vi "S4GUI_001.vi"() -> ()   [LabVIEW 2018] (continued)
            n3129 = call-dynamic "Read State Machine.vi"("error in (no error)"=w7702, "Device in"=w7704) -> ("error out"=w7725:errorcluster, "State Machine.lvclass"=w7726:refnum<class "State Machine.lvclass">, "Device out"=w7722:refnum<class "Channel.lvclass">)  [unwired: 7 in]
            n3130 = call "Next State.vi"("error in (no error)"=w7725, "New_State"=u32 35, "State Machine in"=w7726) -> ("error out"=w7720:errorcluster, "State Machine out"=w7723:refnum<class "State Machine.lvclass">)  [unwired: 7 in]
            n3131 = call-dynamic "Write State Machine.vi"("error in (no error)"=w7720, "State Machine.lvclass"=w7723, "Device in"=w7722) -> ("error out"=w7716:errorcluster, "Device out"=w7715:refnum<class "Channel.lvclass">)  [unwired: 7 in]
            n3132 = call-dynamic "Write Channel.vi"("error in (no error)"=w7716, "Channel.lvclass"=w7715, "Acquisition in"=w7721) -> ("error out"=w7717:errorcluster, "Acquisition out"=w7719:refnum<class "Acquisition.lvclass">)  [unwired: 7 in]
            n3133 = call-dynamic "Write AcquisitionC.vi"("error in (no error)"=w7717, "Acquisition.lvclass"=w7719, "S4ACS_GUI in"=w7718) -> ("error out"=w7712:errorcluster, "S4ACS_GUI out"=w7711:refnum<class "S4GUI.lvclass">)  [unwired: 7 in]
          }
        }
      }
      event "Set Temp 4": Value Change {
        n3134 = event-data() -> ("NewVal"=w7729:bool)  [unwired: 1 in]
        n3135 = case shown="True" w7729 {
          tunnel: w7733 -> [w7735 w7749]
          tunnel: w7732 -> [w7734 w7748]
          tunnel: [w7734 w7747] -> w7731
          tunnel: [w7735 w7746] -> w7730
          frame False {
          }
          frame True {
            n3136 = call-dynamic "Read AcquisitionD.vi"("error in (no error)"=w7748, "S4ACS_GUI in"=w7749) -> ("error out"=w7762:errorcluster, "Acquisition.lvclass"=w7763:refnum<class "Acquisition.lvclass">, "S4ACS_GUI out"=w7753:refnum<class "S4GUI.lvclass">)  [unwired: 7 in]
            n3137 = call-dynamic "Read Channel.vi"("error in (no error)"=w7762, "Acquisition in"=w7763) -> ("error out"=w7744:errorcluster, "Channel.lvclass"=w7745:refnum<class "Channel.lvclass">, "Acquisition out"=w7756:refnum<class "Acquisition.lvclass">)  [unwired: 7 in]
            n3138 = call-dynamic "Read Interface.vi"("error in (no error)"=w7744, "Channel in"=w7745) -> ("error out"=w7742:errorcluster, "Interface.lvclass"=w7743:refnum<class "Interface.lvclass">, "Channel out"=w7740:refnum<class "Channel.lvclass">)  [unwired: 7 in]
            n3139 = call-dynamic "Write Temperature.vi"("error in (no error)"=w7742, "Temperature"="Target Temp 4", "Interface in"=w7743) -> ("error out"=w7738:errorcluster, "Interface out"=w7741:refnum<class "Interface.lvclass">)  [unwired: 7 in]
            n3140 = call-dynamic "Write Interface.vi"("error in (no error)"=w7738, "Interface.lvclass"=w7741, "Channel in"=w7740) -> ("error out"=w7737:errorcluster, "Channel out"=w7739:refnum<class "Channel.lvclass">)  [unwired: 7 in]
            n3141 = call-dynamic "Read State Machine.vi"("error in (no error)"=w7737, "Device in"=w7739) -> ("error out"=w7760:errorcluster, "State Machine.lvclass"=w7761:refnum<class "State Machine.lvclass">, "Device out"=w7757:refnum<class "Channel.lvclass">)  [unwired: 7 in]
            n3142 = call "Next State.vi"("error in (no error)"=w7760, "New_State"=u32 35, "State Machine in"=w7761) -> ("error out"=w7755:errorcluster, "State Machine out"=w7758:refnum<class "State Machine.lvclass">)  [unwired: 7 in]
            n3143 = call-dynamic "Write State Machine.vi"("error in (no error)"=w7755, "State Machine.lvclass"=w7758, "Device in"=w7757) -> ("error out"=w7751:errorcluster, "Device out"=w7750:refnum<class "Channel.lvclass">)  [unwired: 7 in]
            n3144 = call-dynamic "Write Channel.vi"("error in (no error)"=w7751, "Channel.lvclass"=w7750, "Acquisition in"=w7756) -> ("error out"=w7752:errorcluster, "Acquisition out"=w7754:refnum<class "Acquisition.lvclass">)  [unwired: 7 in]
            n3145 = call-dynamic "Write AcquisitionD.vi"("error in (no error)"=w7752, "Acquisition.lvclass"=w7754, "S4ACS_GUI in"=w7753) -> ("error out"=w7747:errorcluster, "S4ACS_GUI out"=w7746:refnum<class "S4GUI.lvclass">)  [unwired: 7 in]
          }
        }
      }
      event "Avança Estado": Value Change {
        n3146 = event-data() -> ()  [unwired: 1 in, 4 out]
        n3147 = call-dynamic "Read Sync Box.lvclass.vi"("error in (no error)"=w7772, "SPARC4_AC in"=w7773) -> ("error out"=w7785:errorcluster, "Sync Box.lvclass"=w7786:refnum<class "Sync Box.lvclass">, "SPARC4_AC out"=w7777:refnum<class "S4GUI.lvclass">)  [unwired: 7 in]
        n3148 = call-dynamic "Read Trigger.lvclass.vi"("error in (no error)"=w7785, "Sync Box in"=w7786) -> ("error out"=w7783:errorcluster, "Trigger.lvclass"=w7784:refnum<class "Trigger.lvclass">, "Sync Box out"=w7780:refnum<class "Sync Box.lvclass">)  [unwired: 7 in]
        n3149 = call-dynamic "Read State Machine.vi"("error in (no error)"=w7783, "Device in"=w7784) -> ("error out"=w7769:errorcluster, "State Machine.lvclass"=w7770:refnum<class "State Machine.lvclass">, "Device out"=w7781:refnum<class "Trigger.lvclass">)  [unwired: 7 in]
        n3150 = call-dynamic "Read State.vi"("error in (no error)"=w7769, "State Machine in"=w7770) -> ("error out"=w7765:errorcluster, "State"=w7768:i32, "State Machine out"=w7766:refnum<class "State Machine.lvclass">)  [unwired: 7 in]
        n3151 = Increment(x=w7768) -> (x+1=w7767:i32)
        n3152 = call "Next State.vi"("error in (no error)"=w7765, "New_State"=w7767, "State Machine in"=w7766) -> ("error out"=w7779:errorcluster, "State Machine out"=w7782:refnum<class "State Machine.lvclass">)  [unwired: 7 in]
        n3153 = call-dynamic "Write State Machine.vi"("error in (no error)"=w7779, "State Machine.lvclass"=w7782, "Device in"=w7781) -> ("error out"=w7775:errorcluster, "Device out"=w7774:refnum<class "Trigger.lvclass">)  [unwired: 7 in]
        n3154 = call-dynamic "Write Trigger.lvclass.vi"("error in (no error)"=w7775, "Trigger.lvclass"=w7774, "Sync Box in"=w7780) -> ("error out"=w7776:errorcluster, "Sync Box out"=w7778:refnum<class "Sync Box.lvclass">)  [unwired: 7 in]
        n3155 = call-dynamic "Write Sync Box.lvclass.vi"("error in (no error)"=w7776, "Sync Box.lvclass"=w7778, "SPARC4_AC in"=w7777) -> ("error out"=w7771:errorcluster, "SPARC4_AC out"=w7764:refnum<class "S4GUI.lvclass">)  [unwired: 7 in]
      }
      event "DelayA": Value Change {
        n3156 = event-data() -> ("NewVal"=w7788:string)  [unwired: 1 in, 3 out]
        n3157 = call-dynamic "Read Sync Box.lvclass.vi"("error in (no error)"=w7792, "SPARC4_AC in"=w7793) -> ("error out"=w7800:errorcluster, "Sync Box.lvclass"=w7801:refnum<class "Sync Box.lvclass">, "SPARC4_AC out"=w7797:refnum<class "S4GUI.lvclass">)  [unwired: 7 in]
        n3158 = call-dynamic "Read Trigger.lvclass.vi"("error in (no error)"=w7800, "Sync Box in"=w7801) -> ("error out"=w7789:errorcluster, "Trigger.lvclass"=w7790:refnum<class "Trigger.lvclass">, "Sync Box out"=w7799:refnum<class "Sync Box.lvclass">)  [unwired: 7 in]
        n3159 = call-dynamic "Write DelayA.vi"("error in (no error)"=w7789, "DelayA"=w7788, "Trigger in"=w7790) -> ("error out"=w7795:errorcluster, "Trigger out"=w7794:refnum<class "Trigger.lvclass">)  [unwired: 7 in]
        n3160 = call-dynamic "Write Trigger.lvclass.vi"("error in (no error)"=w7795, "Trigger.lvclass"=w7794, "Sync Box in"=w7799) -> ("error out"=w7796:errorcluster, "Sync Box out"=w7798:refnum<class "Sync Box.lvclass">)  [unwired: 7 in]
        n3161 = call-dynamic "Write Sync Box.lvclass.vi"("error in (no error)"=w7796, "Sync Box.lvclass"=w7798, "SPARC4_AC in"=w7797) -> ("error out"=w7791:errorcluster, "SPARC4_AC out"=w7787:refnum<class "S4GUI.lvclass">)  [unwired: 7 in]
      }
      event "DelayB": Value Change {
        n3162 = event-data() -> ("NewVal"=w7803:string)  [unwired: 1 in, 3 out]
        n3163 = call-dynamic "Read Sync Box.lvclass.vi"("error in (no error)"=w7807, "SPARC4_AC in"=w7808) -> ("error out"=w7815:errorcluster, "Sync Box.lvclass"=w7816:refnum<class "Sync Box.lvclass">, "SPARC4_AC out"=w7812:refnum<class "S4GUI.lvclass">)  [unwired: 7 in]
        n3164 = call-dynamic "Read Trigger.lvclass.vi"("error in (no error)"=w7815, "Sync Box in"=w7816) -> ("error out"=w7804:errorcluster, "Trigger.lvclass"=w7805:refnum<class "Trigger.lvclass">, "Sync Box out"=w7814:refnum<class "Sync Box.lvclass">)  [unwired: 7 in]
        n3165 = call-dynamic "Write DelayB.vi"("error in (no error)"=w7804, "DelayB"=w7803, "Trigger in"=w7805) -> ("error out"=w7810:errorcluster, "Trigger out"=w7809:refnum<class "Trigger.lvclass">)  [unwired: 7 in]
        n3166 = call-dynamic "Write Trigger.lvclass.vi"("error in (no error)"=w7810, "Trigger.lvclass"=w7809, "Sync Box in"=w7814) -> ("error out"=w7811:errorcluster, "Sync Box out"=w7813:refnum<class "Sync Box.lvclass">)  [unwired: 7 in]
        n3167 = call-dynamic "Write Sync Box.lvclass.vi"("error in (no error)"=w7811, "Sync Box.lvclass"=w7813, "SPARC4_AC in"=w7812) -> ("error out"=w7806:errorcluster, "SPARC4_AC out"=w7802:refnum<class "S4GUI.lvclass">)  [unwired: 7 in]
      }
      event "DelayC": Value Change {
        n3168 = event-data() -> ("NewVal"=w7818:string)  [unwired: 1 in, 3 out]
        n3169 = call-dynamic "Read Sync Box.lvclass.vi"("error in (no error)"=w7822, "SPARC4_AC in"=w7823) -> ("error out"=w7830:errorcluster, "Sync Box.lvclass"=w7831:refnum<class "Sync Box.lvclass">, "SPARC4_AC out"=w7827:refnum<class "S4GUI.lvclass">)  [unwired: 7 in]
        n3170 = call-dynamic "Read Trigger.lvclass.vi"("error in (no error)"=w7830, "Sync Box in"=w7831) -> ("error out"=w7819:errorcluster, "Trigger.lvclass"=w7820:refnum<class "Trigger.lvclass">, "Sync Box out"=w7829:refnum<class "Sync Box.lvclass">)  [unwired: 7 in]
        n3171 = call-dynamic "Write DelayC.vi"("error in (no error)"=w7819, "DelayC"=w7818, "Trigger in"=w7820) -> ("error out"=w7825:errorcluster, "Trigger out"=w7824:refnum<class "Trigger.lvclass">)  [unwired: 7 in]
        n3172 = call-dynamic "Write Trigger.lvclass.vi"("error in (no error)"=w7825, "Trigger.lvclass"=w7824, "Sync Box in"=w7829) -> ("error out"=w7826:errorcluster, "Sync Box out"=w7828:refnum<class "Sync Box.lvclass">)  [unwired: 7 in]
        n3173 = call-dynamic "Write Sync Box.lvclass.vi"("error in (no error)"=w7826, "Sync Box.lvclass"=w7828, "SPARC4_AC in"=w7827) -> ("error out"=w7821:errorcluster, "SPARC4_AC out"=w7817:refnum<class "S4GUI.lvclass">)  [unwired: 7 in]
      }
      event "DelayD": Value Change {
        n3174 = event-data() -> ("NewVal"=w7833:string)  [unwired: 1 in, 3 out]
        n3175 = call-dynamic "Read Sync Box.lvclass.vi"("error in (no error)"=w7837, "SPARC4_AC in"=w7838) -> ("error out"=w7845:errorcluster, "Sync Box.lvclass"=w7846:refnum<class "Sync Box.lvclass">, "SPARC4_AC out"=w7842:refnum<class "S4GUI.lvclass">)  [unwired: 7 in]
        n3176 = call-dynamic "Read Trigger.lvclass.vi"("error in (no error)"=w7845, "Sync Box in"=w7846) -> ("error out"=w7834:errorcluster, "Trigger.lvclass"=w7835:refnum<class "Trigger.lvclass">, "Sync Box out"=w7844:refnum<class "Sync Box.lvclass">)  [unwired: 7 in]
        n3177 = call-dynamic "Write DelayD.vi"("error in (no error)"=w7834, "DelayD"=w7833, "Trigger in"=w7835) -> ("error out"=w7840:errorcluster, "Trigger out"=w7839:refnum<class "Trigger.lvclass">)  [unwired: 7 in]
        n3178 = call-dynamic "Write Trigger.lvclass.vi"("error in (no error)"=w7840, "Trigger.lvclass"=w7839, "Sync Box in"=w7844) -> ("error out"=w7841:errorcluster, "Sync Box out"=w7843:refnum<class "Sync Box.lvclass">)  [unwired: 7 in]
        n3179 = call-dynamic "Write Sync Box.lvclass.vi"("error in (no error)"=w7841, "Sync Box.lvclass"=w7843, "SPARC4_AC in"=w7842) -> ("error out"=w7836:errorcluster, "SPARC4_AC out"=w7832:refnum<class "S4GUI.lvclass">)  [unwired: 7 in]
      }
      event "WidthA": Value Change {
        n3180 = event-data() -> ("NewVal"=w7848:string)  [unwired: 1 in, 3 out]
        n3181 = call-dynamic "Read Sync Box.lvclass.vi"("error in (no error)"=w7852, "SPARC4_AC in"=w7853) -> ("error out"=w7860:errorcluster, "Sync Box.lvclass"=w7861:refnum<class "Sync Box.lvclass">, "SPARC4_AC out"=w7857:refnum<class "S4GUI.lvclass">)  [unwired: 7 in]
        n3182 = call-dynamic "Read Trigger.lvclass.vi"("error in (no error)"=w7860, "Sync Box in"=w7861) -> ("error out"=w7849:errorcluster, "Trigger.lvclass"=w7850:refnum<class "Trigger.lvclass">, "Sync Box out"=w7859:refnum<class "Sync Box.lvclass">)  [unwired: 7 in]
        n3183 = call-dynamic "Write WidthA.vi"("error in (no error)"=w7849, "WidthA"=w7848, "Trigger in"=w7850) -> ("error out"=w7855:errorcluster, "Trigger out"=w7854:refnum<class "Trigger.lvclass">)  [unwired: 7 in]
        n3184 = call-dynamic "Write Trigger.lvclass.vi"("error in (no error)"=w7855, "Trigger.lvclass"=w7854, "Sync Box in"=w7859) -> ("error out"=w7856:errorcluster, "Sync Box out"=w7858:refnum<class "Sync Box.lvclass">)  [unwired: 7 in]
        n3185 = call-dynamic "Write Sync Box.lvclass.vi"("error in (no error)"=w7856, "Sync Box.lvclass"=w7858, "SPARC4_AC in"=w7857) -> ("error out"=w7851:errorcluster, "SPARC4_AC out"=w7847:refnum<class "S4GUI.lvclass">)  [unwired: 7 in]
      }
      event "WidthB": Value Change {
        n3186 = event-data() -> ("NewVal"=w7863:string)  [unwired: 1 in, 3 out]
        n3187 = call-dynamic "Read Sync Box.lvclass.vi"("error in (no error)"=w7867, "SPARC4_AC in"=w7868) -> ("error out"=w7875:errorcluster, "Sync Box.lvclass"=w7876:refnum<class "Sync Box.lvclass">, "SPARC4_AC out"=w7872:refnum<class "S4GUI.lvclass">)  [unwired: 7 in]
        n3188 = call-dynamic "Read Trigger.lvclass.vi"("error in (no error)"=w7875, "Sync Box in"=w7876) -> ("error out"=w7864:errorcluster, "Trigger.lvclass"=w7865:refnum<class "Trigger.lvclass">, "Sync Box out"=w7874:refnum<class "Sync Box.lvclass">)  [unwired: 7 in]
        n3189 = call-dynamic "Write WidthB.vi"("error in (no error)"=w7864, "WidthB"=w7863, "Trigger in"=w7865) -> ("error out"=w7870:errorcluster, "Trigger out"=w7869:refnum<class "Trigger.lvclass">)  [unwired: 7 in]
        n3190 = call-dynamic "Write Trigger.lvclass.vi"("error in (no error)"=w7870, "Trigger.lvclass"=w7869, "Sync Box in"=w7874) -> ("error out"=w7871:errorcluster, "Sync Box out"=w7873:refnum<class "Sync Box.lvclass">)  [unwired: 7 in]
        n3191 = call-dynamic "Write Sync Box.lvclass.vi"("error in (no error)"=w7871, "Sync Box.lvclass"=w7873, "SPARC4_AC in"=w7872) -> ("error out"=w7866:errorcluster, "SPARC4_AC out"=w7862:refnum<class "S4GUI.lvclass">)  [unwired: 7 in]
      }
      event "WidthC": Value Change {
        n3192 = event-data() -> ("NewVal"=w7878:string)  [unwired: 1 in, 3 out]
        n3193 = call-dynamic "Read Sync Box.lvclass.vi"("error in (no error)"=w7882, "SPARC4_AC in"=w7883) -> ("error out"=w7890:errorcluster, "Sync Box.lvclass"=w7891:refnum<class "Sync Box.lvclass">, "SPARC4_AC out"=w7887:refnum<class "S4GUI.lvclass">)  [unwired: 7 in]
        n3194 = call-dynamic "Read Trigger.lvclass.vi"("error in (no error)"=w7890, "Sync Box in"=w7891) -> ("error out"=w7879:errorcluster, "Trigger.lvclass"=w7880:refnum<class "Trigger.lvclass">, "Sync Box out"=w7889:refnum<class "Sync Box.lvclass">)  [unwired: 7 in]
        n3195 = call-dynamic "Write WidthC.vi"("error in (no error)"=w7879, "WidthC"=w7878, "Trigger in"=w7880) -> ("error out"=w7885:errorcluster, "Trigger out"=w7884:refnum<class "Trigger.lvclass">)  [unwired: 7 in]
        n3196 = call-dynamic "Write Trigger.lvclass.vi"("error in (no error)"=w7885, "Trigger.lvclass"=w7884, "Sync Box in"=w7889) -> ("error out"=w7886:errorcluster, "Sync Box out"=w7888:refnum<class "Sync Box.lvclass">)  [unwired: 7 in]
        n3197 = call-dynamic "Write Sync Box.lvclass.vi"("error in (no error)"=w7886, "Sync Box.lvclass"=w7888, "SPARC4_AC in"=w7887) -> ("error out"=w7881:errorcluster, "SPARC4_AC out"=w7877:refnum<class "S4GUI.lvclass">)  [unwired: 7 in]
      }
      event "WidthD": Value Change {
        n3198 = event-data() -> ("NewVal"=w7893:string)  [unwired: 1 in, 3 out]
        n3199 = call-dynamic "Read Sync Box.lvclass.vi"("error in (no error)"=w7897, "SPARC4_AC in"=w7898) -> ("error out"=w7905:errorcluster, "Sync Box.lvclass"=w7906:refnum<class "Sync Box.lvclass">, "SPARC4_AC out"=w7902:refnum<class "S4GUI.lvclass">)  [unwired: 7 in]
        n3200 = call-dynamic "Read Trigger.lvclass.vi"("error in (no error)"=w7905, "Sync Box in"=w7906) -> ("error out"=w7894:errorcluster, "Trigger.lvclass"=w7895:refnum<class "Trigger.lvclass">, "Sync Box out"=w7904:refnum<class "Sync Box.lvclass">)  [unwired: 7 in]
        n3201 = call-dynamic "Write WidthD.vi"("error in (no error)"=w7894, "WidthD"=w7893, "Trigger in"=w7895) -> ("error out"=w7900:errorcluster, "Trigger out"=w7899:refnum<class "Trigger.lvclass">)  [unwired: 7 in]
        n3202 = call-dynamic "Write Trigger.lvclass.vi"("error in (no error)"=w7900, "Trigger.lvclass"=w7899, "Sync Box in"=w7904) -> ("error out"=w7901:errorcluster, "Sync Box out"=w7903:refnum<class "Sync Box.lvclass">)  [unwired: 7 in]
        n3203 = call-dynamic "Write Sync Box.lvclass.vi"("error in (no error)"=w7901, "Sync Box.lvclass"=w7903, "SPARC4_AC in"=w7902) -> ("error out"=w7896:errorcluster, "SPARC4_AC out"=w7892:refnum<class "S4GUI.lvclass">)  [unwired: 7 in]
      }
      event "WPROT_set": Value Change {
        # "Espera até 10 x 1s = 10s\npara condition de WPROT\n ir para READY"
        n3204 = event-data() -> ()  [unwired: 1 in, 4 out]
        n3205 = call "Read Instrument.lvclass.vi"("error in (no error)"=w7928, "S4ACS_GUI in"=w7929) -> ("error out"=w7926:errorcluster, "Instrument.lvclass"=w7927:refnum<class "Instrument.lvclass">, "S4ACS_GUI out"=w7915:refnum<class "S4GUI.lvclass">)  [unwired: 7 in]
        n3206 = call "Read WPROT.vi"("error in (no error)"=w7926, "Instrument in"=w7927) -> ("error out"=w7922:errorcluster, "Opt_Selector.lvclass"=w7925:refnum<class "Opt_Selector.lvclass">, "Instrument out"=w7918:refnum<class "Instrument.lvclass">)  [unwired: 7 in]
        n3207 = call-dynamic "Read State Machine.vi"("error in (no error)"=w7922, "Device in"=w7925) -> ("error out"=w7921:errorcluster, "State Machine.lvclass"=w7924:refnum<class "State Machine.lvclass">, "Device out"=w7920:refnum<class "Opt_Selector.lvclass">)  [unwired: 7 in]
        n3208 = call "Next State.vi"("error in (no error)"=w7921, "New_State"=1, "State Machine in"=w7924) -> ("error out"=w7909:errorcluster, "State Machine out"=w7911:refnum<class "State Machine.lvclass">)  [unwired: 7 in]
        n3209 = call-dynamic "Write Timer.vi"("error in (no error)"=w7909, "Timer"=u32 10, "State Machine in"=w7911) -> ("error out"=w7908:errorcluster, "State Machine out"=w7910:refnum<class "State Machine.lvclass">)  [unwired: 7 in]
        n3210 = call-dynamic "Write State Machine.vi"("error in (no error)"=w7908, "State Machine.lvclass"=w7910, "Device in"=w7920) -> ("error out"=w7917:errorcluster, "Device out"=w7919:refnum<class "Opt_Selector.lvclass">)  [unwired: 7 in]
        n3211 = call "Write WPROT.vi"("error in (no error)"=w7917, "Opt_Selector.lvclass"=w7919, "Instrument in"=w7918) -> ("error out"=w7914:errorcluster, "Instrument out"=w7916:refnum<class "Instrument.lvclass">)  [unwired: 7 in]
        n3212 = call "Write Instrument.lvclass.vi"("error in (no error)"=w7914, "Instrument.lvclass"=w7916, "S4ACS_GUI in"=w7915) -> ("error out"=w7913:errorcluster, "S4ACS_GUI out"=w7912:refnum<class "S4GUI.lvclass">)  [unwired: 7 in]
      }
      event "TARGET NAME WPROT": Value Change {
        n3213 = event-data() -> ()  [unwired: 1 in, 1 out]
        n3214 = property on="TARGET NAME WPROT" class="Enum (strict)"() -> ("RingText.Text"=w7956:string)  [unwired: 2 in, 2 out]
        n3215 = call "Read Instrument.lvclass.vi"("error in (no error)"=w7957, "S4ACS_GUI in"=w7958) -> ("error out"=w7965:errorcluster, "Instrument.lvclass"=w7966:refnum<class "Instrument.lvclass">, "S4ACS_GUI out"=w7960:refnum<class "S4GUI.lvclass">)  [unwired: 7 in]
        n3216 = Build Array(-1.0 ("element"), 0.0 ("element"), 22.5 ("element"), 45.0 ("element"), 67.5 ("element"), 90.0 ("element"), 112.5 ("element"), 135.0 ("element"), 157.5 ("element"), 180.0 ("element"), 202.5 ("element"), 225.0 ("element"), 247.5 ("element"), 270.0 ("element"), 292.5 ("element"), 315.0 ("element"), 337.5 ("element")) -> (w7948:dbl[])
        n3217 = call "Read WPROT.vi"("error in (no error)"=w7965, "Instrument in"=w7966) -> ("error out"=w7963:errorcluster, "Opt_Selector.lvclass"=w7964:refnum<class "Opt_Selector.lvclass">, "Instrument out"=w7962:refnum<class "Instrument.lvclass">)  [unwired: 7 in]
        n3218 = call "Write target name.vi"("error in (no error)"=w7963, "target name"=w7956, "Optics in"=w7964) -> ("error out"=w7944:errorcluster, "Optics out"=w7945:refnum<class "Opt_Selector.lvclass">)  [unwired: 7 in]
        n3219 = Index Array(array=w7948, index="TARGET NAME WPROT") -> (element=w7946:dbl)
        n3220 = call "Write target.vi"("error in (no error)"=w7944, "target"=w7946, "Optics in"=w7945) -> ("error out"=w7943:errorcluster, "Optics out"=w7942:refnum<class "Opt_Selector.lvclass">)  [unwired: 7 in]
        n3221 = call "Write WPROT.vi"("error in (no error)"=w7943, "Opt_Selector.lvclass"=w7942, "Instrument in"=w7962) -> ("error out"=w7959:errorcluster, "Instrument out"=w7961:refnum<class "Instrument.lvclass">)  [unwired: 7 in]
        n3222 = call "Write Instrument.lvclass.vi"("error in (no error)"=w7959, "Instrument.lvclass"=w7961, "S4ACS_GUI in"=w7960) -> ("error out"=w7955:errorcluster, "S4ACS_GUI out"=w7930:refnum<class "S4GUI.lvclass">)  [unwired: 7 in]
      }
      event "TARGET NAME WPSEL": Value Change {
        n3223 = event-data() -> ()  [unwired: 1 in, 1 out]
        n3224 = property on="TARGET NAME WPSEL" class="Enum (strict)"() -> ("RingText.Text"=w7968:string)  [unwired: 2 in, 2 out]
        n3225 = call "Read Instrument.lvclass.vi"("error in (no error)"=w7981, "S4ACS_GUI in"=w7982) -> ("error out"=w7989:errorcluster, "Instrument.lvclass"=w7990:refnum<class "Instrument.lvclass">, "S4ACS_GUI out"=w7984:refnum<class "S4GUI.lvclass">)  [unwired: 7 in]
        n3226 = Build Array(-1.0 ("element"), 80.0 ("element"), 0.0 ("element"), 160.0 ("element")) -> (w7975:dbl[])
        n3227 = call "Read WPSEL.vi"("error in (no error)"=w7989, "Instrument in"=w7990) -> ("error out"=w7987:errorcluster, "Opt_Selector.lvclass"=w7988:refnum<class "Opt_Selector.lvclass">, "Instrument out"=w7986:refnum<class "Instrument.lvclass">)  [unwired: 7 in]
        n3228 = call "Write target name.vi"("error in (no error)"=w7987, "target name"=w7968, "Optics in"=w7988) -> ("error out"=w7972:errorcluster, "Optics out"=w7973:refnum<class "Opt_Selector.lvclass">)  [unwired: 7 in]
        n3229 = Index Array(array=w7975, index="TARGET NAME WPSEL") -> (element=w7974:dbl)
        n3230 = call "Write target.vi"("error in (no error)"=w7972, "target"=w7974, "Optics in"=w7973) -> ("error out"=w7971:errorcluster, "Optics out"=w7970:refnum<class "Opt_Selector.lvclass">)  [unwired: 7 in]
        n3231 = call "Write WPSEL.vi"("error in (no error)"=w7971, "Opt_Selector.lvclass"=w7970, "Instrument in"=w7986) -> ("error out"=w7983:errorcluster, "Instrument out"=w7985:refnum<class "Instrument.lvclass">)  [unwired: 7 in]
        n3232 = call "Write Instrument.lvclass.vi"("error in (no error)"=w7983, "Instrument.lvclass"=w7985, "S4ACS_GUI in"=w7984) -> ("error out"=w7980:errorcluster, "S4ACS_GUI out"=w7967:refnum<class "S4GUI.lvclass">)  [unwired: 7 in]
      }
      event "Lambda Selector": Value Change {
        n3233 = event-data() -> ("NewVal"=w7992:u16)  [unwired: 1 in, 1 out]
        n3234 = property on="Lambda Selector" class="Ring (strict)"() -> ("RingText.Text"=w7998:string)  [unwired: 2 in, 2 out]
        n3235 = call "Read Instrument.lvclass.vi"("error in (no error)"=w8023, "S4ACS_GUI in"=w8024) -> ("error out"=w8025:errorcluster, "Instrument.lvclass"=w8000:refnum<class "Instrument.lvclass">, "S4ACS_GUI out"=w7997:refnum<class "S4GUI.lvclass">)  [unwired: 7 in]
        n3236 = Build Array(80.0 ("element"), 0.0 ("element"), 160.0 ("element")) -> (w8018:dbl[])
        n3237 = call "Read WPSEL.vi"("error in (no error)"=w8025, "Instrument in"=w8000) -> ("error out"=w8007:errorcluster, "Opt_Selector.lvclass"=w8006:refnum<class "Opt_Selector.lvclass">, "Instrument out"=w7999:refnum<class "Instrument.lvclass">)  [unwired: 7 in]
        n3238 = Index Array(array=w8018, index=w7992) -> (element=w8017:dbl)
        n3239 = call "Write target.vi"("error in (no error)"=w8007, "target"=w8017, "Optics in"=w8006) -> ("error out"=w8004:errorcluster, "Optics out"=w8005:refnum<class "Opt_Selector.lvclass">)  [unwired: 7 in]
        n3240 = case shown="\"Lambda/2\"" w7998 {
          selector: w7998 -> [w8028 _ _]
          tunnel: [w8028 "ON" "ON"] -> w8009
          tunnel: [0.0 ("element") 30.0 ("element") 30.0 ("element")] -> w8008
          tunnel: [w8028 "L/2" "L/4"] -> w8001
          frame "OFF", Default {
            n3241 = property on="Calibrator Selector" class="Ring (strict)"("DisabledEnum"=T7."Disabled and Grayed Out" ("Disabled")) -> ()  [unwired: 2 in, 2 out]
          }
          frame "Lambda/2" {
            n3242 = property on="Calibrator Selector" class="Ring (strict)"("DisabledEnum"=T7."Enabled" ("Disabled")) -> ()  [unwired: 2 in, 2 out]
          }
          frame "Lambda/4" {
            n3243 = property on="Calibrator Selector" class="Ring (strict)"("DisabledEnum"=T7."Enabled" ("Disabled")) -> ()  [unwired: 2 in, 2 out]
          }
        }
        n3244 = call "Write target name.vi"("error in (no error)"=w8004, "target name"=w8001, "Optics in"=w8005) -> ("error out"=w8003:errorcluster, "Optics out"=w8002:refnum<class "Opt_Selector.lvclass">)  [unwired: 7 in]
        n3245 = call "Write WPSEL.vi"("error in (no error)"=w8003, "Opt_Selector.lvclass"=w8002, "Instrument in"=w7999) -> ("error out"=w7994:errorcluster, "Instrument out"=w7993:refnum<class "Instrument.lvclass">)  [unwired: 7 in]
        n3246 = call "Read ASEL.vi"("error in (no error)"=w7994, "Instrument in"=w7993) -> ("error out"=w8014:errorcluster, "Opt_Selector.lvclass"=w8012:refnum<class "Opt_Selector.lvclass">, "Instrument out"=w7996:refnum<class "Instrument.lvclass">)  [unwired: 7 in]
        n3247 = call "Write target name.vi"("error in (no error)"=w8014, "target name"=w8009, "Optics in"=w8012) -> ("error out"=w8015:errorcluster, "Optics out"=w8011:refnum<class "Opt_Selector.lvclass">)  [unwired: 7 in]
        n3248 = call "Write target.vi"("error in (no error)"=w8015, "target"=w8008, "Optics in"=w8011) -> ("error out"=w8016:errorcluster, "Optics out"=w8010:refnum<class "Opt_Selector.lvclass">)  [unwired: 7 in]
        n3249 = call "Write ASEL.vi"("error in (no error)"=w8016, "Opt_Selector.lvclass"=w8010, "Instrument in"=w7996) -> ("error out"=w8013:errorcluster, "Instrument out"=w7995:refnum<class "Instrument.lvclass">)  [unwired: 7 in]
        n3250 = call "Write Instrument.lvclass.vi"("error in (no error)"=w8013, "Instrument.lvclass"=w7995, "S4ACS_GUI in"=w7997) -> ("error out"=w8022:errorcluster, "S4ACS_GUI out"=w7991:refnum<class "S4GUI.lvclass">)  [unwired: 7 in]
      }
      event "Calibrator Selector": Value Change {
        n3251 = event-data() -> ()  [unwired: 1 in, 6 out]
        n3252 = call "Read Instrument.lvclass.vi"("error in (no error)"=w8057, "S4ACS_GUI in"=w8058) -> ("error out"=w8061:errorcluster, "Instrument.lvclass"=w8062:refnum<class "Instrument.lvclass">, "S4ACS_GUI out"=w8059:refnum<class "S4GUI.lvclass">)  [unwired: 7 in]
        n3253 = property on="Calibrator Selector" class="Ring (strict)"() -> ("RingText.Text"=w8043:string)  [unwired: 2 in, 2 out]
        n3254 = Build Array(0.0 ("element"), 72.0 ("element"), 144.0 ("element"), 216.0 ("element"), 288.0 ("element")) -> (w8052:dbl[])
        n3255 = call "Read CALW.vi"("error in (no error)"=w8061, "Instrument in"=w8062) -> ("error out"=w8050:errorcluster, "Opt_Selector.lvclass"=w8049:refnum<class "Opt_Selector.lvclass">, "Instrument out"=w8060:refnum<class "Instrument.lvclass">)  [unwired: 7 in]
        n3256 = Index Array(array=w8052, index="Calibrator Selector") -> (element=w8051:dbl)
        n3257 = call "Write target.vi"("error in (no error)"=w8050, "target"=w8051, "Optics in"=w8049) -> ("error out"=w8047:errorcluster, "Optics out"=w8048:refnum<class "Opt_Selector.lvclass">)  [unwired: 7 in]
        n3258 = case shown="\"POLARIZER\"" w8043 {
          selector: w8043 -> [_ w8064 w8065 w8066 w8067]
          tunnel: ["OFF" w8064 w8065 w8066 w8067] -> w8044
          frame "OFF", Default {
          }
          frame "POLARIZER" {
          }
          frame "DEPOLARIZER" {
          }
          frame "PINHOLE" {
          }
          frame "SHUTTER" {
          }
        }
        n3259 = call "Write target name.vi"("error in (no error)"=w8047, "target name"=w8044, "Optics in"=w8048) -> ("error out"=w8046:errorcluster, "Optics out"=w8045:refnum<class "Opt_Selector.lvclass">)  [unwired: 7 in]
        n3260 = call "Write CALW.vi"("error in (no error)"=w8046, "Opt_Selector.lvclass"=w8045, "Instrument in"=w8060) -> ("error out"=w8040:errorcluster, "Instrument out"=w8041:refnum<class "Instrument.lvclass">)  [unwired: 7 in]
        n3261 = call "Write Instrument.lvclass.vi"("error in (no error)"=w8040, "Instrument.lvclass"=w8041, "S4ACS_GUI in"=w8059) -> ("error out"=w8056:errorcluster, "S4ACS_GUI out"=w8039:refnum<class "S4GUI.lvclass">)  [unwired: 7 in]
      }
      event "TARGET NAME CALW": Value Change {
        # "aqui também"
        # "aqui também"
        # "OV20230426: Montagem do CALW\nestá POL e DEPOL invertidos"
        n3262 = event-data() -> ()  [unwired: 1 in, 6 out]
        n3263 = property on="TARGET NAME CALW" class="Enum (strict)"() -> ("RingText.Text"=w8069:string)  [unwired: 2 in, 2 out]
        n3264 = case shown="Default" w8069 {
          selector: w8069 -> [_ _ w8097]
          tunnel: ["DEPOLARIZER" "POLARIZER" w8097] -> w8068
          frame "POLARIZER" {
          }
          frame "DEPOLARIZER" {
          }
          frame Default {
          }
        }
        n3265 = call "Read Instrument.lvclass.vi"("error in (no error)"=w8085, "S4ACS_GUI in"=w8086) -> ("error out"=w8093:errorcluster, "Instrument.lvclass"=w8094:refnum<class "Instrument.lvclass">, "S4ACS_GUI out"=w8088:refnum<class "S4GUI.lvclass">)  [unwired: 7 in]
        n3266 = Build Array(-1.0 ("element"), 0.0 ("element"), 288.0 ("element"), 144.0 ("element"), 216.0 ("element"), 72.0 ("element")) -> (w8079:dbl[])
        n3267 = call "Read CALW.vi"("error in (no error)"=w8093, "Instrument in"=w8094) -> ("error out"=w8091:errorcluster, "Opt_Selector.lvclass"=w8092:refnum<class "Opt_Selector.lvclass">, "Instrument out"=w8090:refnum<class "Instrument.lvclass">)  [unwired: 7 in]
        n3268 = call "Write target name.vi"("error in (no error)"=w8091, "target name"=w8068, "Optics in"=w8092) -> ("error out"=w8076:errorcluster, "Optics out"=w8077:refnum<class "Opt_Selector.lvclass">)  [unwired: 7 in]
        n3269 = Index Array(array=w8079, index="TARGET NAME CALW") -> (element=w8078:dbl)
        n3270 = call "Write target.vi"("error in (no error)"=w8076, "target"=w8078, "Optics in"=w8077) -> ("error out"=w8075:errorcluster, "Optics out"=w8074:refnum<class "Opt_Selector.lvclass">)  [unwired: 7 in]
        n3271 = call "Write CALW.vi"("error in (no error)"=w8075, "Opt_Selector.lvclass"=w8074, "Instrument in"=w8090) -> ("error out"=w8087:errorcluster, "Instrument out"=w8089:refnum<class "Instrument.lvclass">)  [unwired: 7 in]
        n3272 = call "Write Instrument.lvclass.vi"("error in (no error)"=w8087, "Instrument.lvclass"=w8089, "S4ACS_GUI in"=w8088) -> ("error out"=w8084:errorcluster, "S4ACS_GUI out"=w8070:refnum<class "S4GUI.lvclass">)  [unwired: 7 in]
      }
      event "TARGET NAME ASEL": Value Change {
        n3273 = event-data() -> ()  [unwired: 1 in, 6 out]
        n3274 = property on="TARGET NAME ASEL" class="Enum (strict)"() -> ("RingText.Text"=w8100:string)  [unwired: 2 in, 2 out]
        n3275 = call "Read Instrument.lvclass.vi"("error in (no error)"=w8111, "S4ACS_GUI in"=w8112) -> ("error out"=w8119:errorcluster, "Instrument.lvclass"=w8120:refnum<class "Instrument.lvclass">, "S4ACS_GUI out"=w8114:refnum<class "S4GUI.lvclass">)  [unwired: 7 in]
        n3276 = Build Array(-1.0 ("element"), 0.0 ("element"), 30.0 ("element")) -> (w8106:dbl[])
        n3277 = call "Read ASEL.vi"("error in (no error)"=w8119, "Instrument in"=w8120) -> ("error out"=w8117:errorcluster, "Opt_Selector.lvclass"=w8118:refnum<class "Opt_Selector.lvclass">, "Instrument out"=w8116:refnum<class "Instrument.lvclass">)  [unwired: 7 in]
        n3278 = call "Write target name.vi"("error in (no error)"=w8117, "target name"=w8100, "Optics in"=w8118) -> ("error out"=w8103:errorcluster, "Optics out"=w8104:refnum<class "Opt_Selector.lvclass">)  [unwired: 7 in]
        n3279 = Index Array(array=w8106, index="TARGET NAME ASEL") -> (element=w8105:dbl)
        n3280 = call "Write target.vi"("error in (no error)"=w8103, "target"=w8105, "Optics in"=w8104) -> ("error out"=w8102:errorcluster, "Optics out"=w8101:refnum<class "Opt_Selector.lvclass">)  [unwired: 7 in]
        n3281 = call "Write ASEL.vi"("error in (no error)"=w8102, "Opt_Selector.lvclass"=w8101, "Instrument in"=w8116) -> ("error out"=w8113:errorcluster, "Instrument out"=w8115:refnum<class "Instrument.lvclass">)  [unwired: 7 in]
        n3282 = call "Write Instrument.lvclass.vi"("error in (no error)"=w8113, "Instrument.lvclass"=w8115, "S4ACS_GUI in"=w8114) -> ("error out"=w8110:errorcluster, "S4ACS_GUI out"=w8098:refnum<class "S4GUI.lvclass">)  [unwired: 7 in]
      }
      event "WPROT_stop": Value Change {
        n3283 = event-data() -> ()  [unwired: 1 in, 4 out]
        n3284 = call "Read Instrument.lvclass.vi"("error in (no error)"=w8139, "S4ACS_GUI in"=w8140) -> ("error out"=w8137:errorcluster, "Instrument.lvclass"=w8138:refnum<class "Instrument.lvclass">, "S4ACS_GUI out"=w8124:refnum<class "S4GUI.lvclass">)  [unwired: 7 in]
        n3285 = call "Read WPROT.vi"("error in (no error)"=w8137, "Instrument in"=w8138) -> ("error out"=w8133:errorcluster, "Opt_Selector.lvclass"=w8136:refnum<class "Opt_Selector.lvclass">, "Instrument out"=w8127:refnum<class "Instrument.lvclass">)  [unwired: 7 in]
        n3286 = call-dynamic "Read State Machine.vi"("error in (no error)"=w8133, "Device in"=w8136) -> ("error out"=w8132:errorcluster, "State Machine.lvclass"=w8135:refnum<class "State Machine.lvclass">, "Device out"=w8129:refnum<class "Opt_Selector.lvclass">)  [unwired: 7 in]
        n3287 = call "Next State.vi"("error in (no error)"=w8132, "New_State"=10, "State Machine in"=w8135) -> ("error out"=w8131:errorcluster, "State Machine out"=w8130:refnum<class "State Machine.lvclass">)  [unwired: 7 in]
        n3288 = call-dynamic "Write State Machine.vi"("error in (no error)"=w8131, "State Machine.lvclass"=w8130, "Device in"=w8129) -> ("error out"=w8126:errorcluster, "Device out"=w8128:refnum<class "Opt_Selector.lvclass">)  [unwired: 7 in]
        n3289 = call "Write WPROT.vi"("error in (no error)"=w8126, "Opt_Selector.lvclass"=w8128, "Instrument in"=w8127) -> ("error out"=w8123:errorcluster, "Instrument out"=w8125:refnum<class "Instrument.lvclass">)  [unwired: 7 in]
        n3290 = call "Write Instrument.lvclass.vi"("error in (no error)"=w8123, "Instrument.lvclass"=w8125, "S4ACS_GUI in"=w8124) -> ("error out"=w8122:errorcluster, "S4ACS_GUI out"=w8121:refnum<class "S4GUI.lvclass">)  [unwired: 7 in]
      }
      event "WPROT_init": Value Change {
        n3291 = event-data() -> ()  [unwired: 1 in, 4 out]
        n3292 = call "Read Instrument.lvclass.vi"("error in (no error)"=w8159, "S4ACS_GUI in"=w8160) -> ("error out"=w8157:errorcluster, "Instrument.lvclass"=w8158:refnum<class "Instrument.lvclass">, "S4ACS_GUI out"=w8144:refnum<class "S4GUI.lvclass">)  [unwired: 7 in]
        n3293 = call "Read WPROT.vi"("error in (no error)"=w8157, "Instrument in"=w8158) -> ("error out"=w8153:errorcluster, "Opt_Selector.lvclass"=w8156:refnum<class "Opt_Selector.lvclass">, "Instrument out"=w8147:refnum<class "Instrument.lvclass">)  [unwired: 7 in]
        n3294 = call-dynamic "Read State Machine.vi"("error in (no error)"=w8153, "Device in"=w8156) -> ("error out"=w8152:errorcluster, "State Machine.lvclass"=w8155:refnum<class "State Machine.lvclass">, "Device out"=w8149:refnum<class "Opt_Selector.lvclass">)  [unwired: 7 in]
        n3295 = call "Next State.vi"("error in (no error)"=w8152, "New_State"=30, "State Machine in"=w8155) -> ("error out"=w8151:errorcluster, "State Machine out"=w8150:refnum<class "State Machine.lvclass">)  [unwired: 7 in]
        n3296 = call-dynamic "Write State Machine.vi"("error in (no error)"=w8151, "State Machine.lvclass"=w8150, "Device in"=w8149) -> ("error out"=w8146:errorcluster, "Device out"=w8148:refnum<class "Opt_Selector.lvclass">)  [unwired: 7 in]
        n3297 = call "Write WPROT.vi"("error in (no error)"=w8146, "Opt_Selector.lvclass"=w8148, "Instrument in"=w8147) -> ("error out"=w8143:errorcluster, "Instrument out"=w8145:refnum<class "Instrument.lvclass">)  [unwired: 7 in]
        n3298 = call "Write Instrument.lvclass.vi"("error in (no error)"=w8143, "Instrument.lvclass"=w8145, "S4ACS_GUI in"=w8144) -> ("error out"=w8142:errorcluster, "S4ACS_GUI out"=w8141:refnum<class "S4GUI.lvclass">)  [unwired: 7 in]
      }
      event "WPSEL_target": Value Change {
        n3299 = event-data() -> ("NewVal"=w8170:dbl)  [unwired: 1 in, 3 out]
        n3300 = call "Read Instrument.lvclass.vi"("error in (no error)"=w8174, "S4ACS_GUI in"=w8175) -> ("error out"=w8172:errorcluster, "Instrument.lvclass"=w8173:refnum<class "Instrument.lvclass">, "S4ACS_GUI out"=w8164:refnum<class "S4GUI.lvclass">)  [unwired: 7 in]
        n3301 = call "Read WPSEL.vi"("error in (no error)"=w8172, "Instrument in"=w8173) -> ("error out"=w8169:errorcluster, "Opt_Selector.lvclass"=w8171:refnum<class "Opt_Selector.lvclass">, "Instrument out"=w8167:refnum<class "Instrument.lvclass">)  [unwired: 7 in]
        n3302 = call "Write target.vi"("error in (no error)"=w8169, "target"=w8170, "Optics in"=w8171) -> ("error out"=w8166:errorcluster, "Optics out"=w8168:refnum<class "Opt_Selector.lvclass">)  [unwired: 7 in]
        n3303 = call "Write WPSEL.vi"("error in (no error)"=w8166, "Opt_Selector.lvclass"=w8168, "Instrument in"=w8167) -> ("error out"=w8163:errorcluster, "Instrument out"=w8165:refnum<class "Instrument.lvclass">)  [unwired: 7 in]
        n3304 = call "Write Instrument.lvclass.vi"("error in (no error)"=w8163, "Instrument.lvclass"=w8165, "S4ACS_GUI in"=w8164) -> ("error out"=w8162:errorcluster, "S4ACS_GUI out"=w8161:refnum<class "S4GUI.lvclass">)  [unwired: 7 in]
      }
      event "WPSEL_set": Value Change {
        n3305 = event-data() -> ()  [unwired: 1 in, 4 out]
        n3306 = call "Read Instrument.lvclass.vi"("error in (no error)"=w8194, "S4ACS_GUI in"=w8195) -> ("error out"=w8192:errorcluster, "Instrument.lvclass"=w8193:refnum<class "Instrument.lvclass">, "S4ACS_GUI out"=w8180:refnum<class "S4GUI.lvclass">)  [unwired: 7 in]
        n3307 = call "Read WPSEL.vi"("error in (no error)"=w8192, "Instrument in"=w8193) -> ("error out"=w8189:errorcluster, "Opt_Selector.lvclass"=w8191:refnum<class "Opt_Selector.lvclass">, "Instrument out"=w8183:refnum<class "Instrument.lvclass">)  [unwired: 7 in]
        n3308 = call-dynamic "Read State Machine.vi"("error in (no error)"=w8189, "Device in"=w8191) -> ("error out"=w8188:errorcluster, "State Machine.lvclass"=w8177:refnum<class "State Machine.lvclass">, "Device out"=w8185:refnum<class "Opt_Selector.lvclass">)  [unwired: 7 in]
        n3309 = call "Next State.vi"("error in (no error)"=w8188, "New_State"=1, "State Machine in"=w8177) -> ("error out"=w8187:errorcluster, "State Machine out"=w8186:refnum<class "State Machine.lvclass">)  [unwired: 7 in]
        n3310 = call-dynamic "Write State Machine.vi"("error in (no error)"=w8187, "State Machine.lvclass"=w8186, "Device in"=w8185) -> ("error out"=w8182:errorcluster, "Device out"=w8184:refnum<class "Opt_Selector.lvclass">)  [unwired: 7 in]
        n3311 = call "Write WPSEL.vi"("error in (no error)"=w8182, "Opt_Selector.lvclass"=w8184, "Instrument in"=w8183) -> ("error out"=w8179:errorcluster, "Instrument out"=w8181:refnum<class "Instrument.lvclass">)  [unwired: 7 in]
        n3312 = call "Write Instrument.lvclass.vi"("error in (no error)"=w8179, "Instrument.lvclass"=w8181, "S4ACS_GUI in"=w8180) -> ("error out"=w8178:errorcluster, "S4ACS_GUI out"=w8176:refnum<class "S4GUI.lvclass">)  [unwired: 7 in]
      }
      event "Set Waveplate": Value Change {
        # "Garantir que, quando em POLARIMETRIA, pelo menos WP1 esteja selecionado."
        # "aqui também"
        # "OV20230426: Montagem do CALW\nestá com POL e DEPOL invertidos"
        n3313 = event-data() -> ()  [unwired: 1 in, 4 out]
        n3314 = local read "Calibrator Selector"() -> (w8267:u16)
        n3315 = call "Read Instrument.lvclass.vi"("error in (no error)"=w8265, "S4ACS_GUI in"=w8264) -> ("error out"=w8284:errorcluster, "Instrument.lvclass"=w8285:refnum<class "Instrument.lvclass">, "S4ACS_GUI out"=w8282:refnum<class "S4GUI.lvclass">)  [unwired: 7 in]
        n3316 = property on="Calibrator Selector" class="Ring (strict)"() -> ("RingText.Text"=w8266:string)  [unwired: 2 in, 2 out]
        n3317 = property on="Lambda Selector" class="Ring (strict)"() -> ("RingText.Text"=w8287:string)  [unwired: 2 in, 2 out]
        n3318 = Build Array(0.0 ("element"), 288.0 ("element"), 144.0 ("element"), 216.0 ("element"), 72.0 ("element")) -> (w8278:dbl[])
        n3319 = local read "Lambda Selector"() -> (w8286:u16)
        n3320 = call "Read CALW.vi"("error in (no error)"=w8284, "Instrument in"=w8285) -> ("error out"=w8276:errorcluster, "Opt_Selector.lvclass"=w8275:refnum<class "Opt_Selector.lvclass">, "Instrument out"=w8283:refnum<class "Instrument.lvclass">)  [unwired: 7 in]
        n3321 = Index Array(array=w8278, index=w8267) -> (element=w8277:dbl)
        n3322 = Build Array(80.0 ("element"), 0.0 ("element"), 160.0 ("element")) -> (w8314:dbl[])
        n3323 = call "Write target.vi"("error in (no error)"=w8276, "target"=w8277, "Optics in"=w8275) -> ("error out"=w8273:errorcluster, "Optics out"=w8274:refnum<class "Opt_Selector.lvclass">)  [unwired: 7 in]
        n3324 = case shown="\"DEPOLARIZER\"" w8266 {
          tunnel: ["OFF" w8543 "PINHOLE" "SHUTTER" w8548] -> w8270
          frame "OFF", Default {
          }
          frame "POLARIZER" {
            n3325 = disable-structure shown="Enabled" {
              disable-tunnel: ["POLARIZER" "DEPOLARIZER"] -> w8543
              frame Disabled {
              }
              frame Enabled {
                # "OV20230426: Montagem do CALW\nestá com POL e DEPOL invertidos"
              }
            }
          }
          frame "PINHOLE" {
          }
          frame "SHUTTER" {
          }
          frame "DEPOLARIZER" {
            n3326 = disable-structure shown="Enabled" {
              disable-tunnel: ["POLARIZER" "DEPOLARIZER"] -> w8548
              frame Enabled {
                # "OV20230426: Montagem do CALW\nestá com POL e DEPOL invertidos"
              }
              frame Disabled {
              }
            }
          }
        }
        n3327 = Index Array(array=w8314, index=w8286) -> (element=w8313:dbl)
        n3328 = case shown="\"OFF\", Default" w8287 {
          tunnel: [w8551 "ON" "ON"] -> w8305
          tunnel: [0.0 ("element") 30.0 ("element") 30.0 ("element")] -> w8304
          tunnel: [w8551 "L/2" "L/4"] -> w8297
          frame "OFF", Default {
            w8551 = "OFF"
          }
          frame "Lambda/2" {
          }
          frame "Lambda/4" {
          }
        }
        n3329 = call "Write target name.vi"("error in (no error)"=w8273, "target name"=w8270, "Optics in"=w8274) -> ("error out"=w8272:errorcluster, "Optics out"=w8271:refnum<class "Opt_Selector.lvclass">)  [unwired: 7 in]
        n3330 = call "Write CALW.vi"("error in (no error)"=w8272, "Opt_Selector.lvclass"=w8271, "Instrument in"=w8283) -> ("error out"=w8268:errorcluster, "Instrument out"=w8269:refnum<class "Instrument.lvclass">)  [unwired: 7 in]
        n3331 = call "Write Instrument.lvclass.vi"("error in (no error)"=w8268, "Instrument.lvclass"=w8269, "S4ACS_GUI in"=w8282) -> ("error out"=w8262:errorcluster, "S4ACS_GUI out"=w8263:refnum<class "S4GUI.lvclass">)  [unwired: 7 in]
        n3332 = call "Read Instrument.lvclass.vi"("error in (no error)"=w8262, "S4ACS_GUI in"=w8263) -> ("error out"=w8318:errorcluster, "Instrument.lvclass"=w8296:refnum<class "Instrument.lvclass">, "S4ACS_GUI out"=w8294:refnum<class "S4GUI.lvclass">)  [unwired: 7 in]
        n3333 = call "Read WPSEL.vi"("error in (no error)"=w8318, "Instrument in"=w8296) -> ("error out"=w8303:errorcluster, "Opt_Selector.lvclass"=w8302:refnum<class "Opt_Selector.lvclass">, "Instrument out"=w8295:refnum<class "Instrument.lvclass">)  [unwired: 7 in]
        n3334 = call "Write target.vi"("error in (no error)"=w8303, "target"=w8313, "Optics in"=w8302) -> ("error out"=w8300:errorcluster, "Optics out"=w8301:refnum<class "Opt_Selector.lvclass">)  [unwired: 7 in]
        n3335 = call "Write target name.vi"("error in (no error)"=w8300, "target name"=w8297, "Optics in"=w8301) -> ("error out"=w8299:errorcluster, "Optics out"=w8298:refnum<class "Opt_Selector.lvclass">)  [unwired: 7 in]
        n3336 = call "Write WPSEL.vi"("error in (no error)"=w8299, "Opt_Selector.lvclass"=w8298, "Instrument in"=w8295) -> ("error out"=w8291:errorcluster, "Instrument out"=w8290:refnum<class "Instrument.lvclass">)  [unwired: 7 in]
        n3337 = call "Read ASEL.vi"("error in (no error)"=w8291, "Instrument in"=w8290) -> ("error out"=w8310:errorcluster, "Opt_Selector.lvclass"=w8308:refnum<class "Opt_Selector.lvclass">, "Instrument out"=w8293:refnum<class "Instrument.lvclass">)  [unwired: 7 in]
        n3338 = call "Write target name.vi"("error in (no error)"=w8310, "target name"=w8305, "Optics in"=w8308) -> ("error out"=w8311:errorcluster, "Optics out"=w8307:refnum<class "Opt_Selector.lvclass">)  [unwired: 7 in]
        n3339 = call "Write target.vi"("error in (no error)"=w8311, "target"=w8304, "Optics in"=w8307) -> ("error out"=w8312:errorcluster, "Optics out"=w8306:refnum<class "Opt_Selector.lvclass">)  [unwired: 7 in]
        n3340 = call "Write ASEL.vi"("error in (no error)"=w8312, "Opt_Selector.lvclass"=w8306, "Instrument in"=w8293) -> ("error out"=w8309:errorcluster, "Instrument out"=w8292:refnum<class "Instrument.lvclass">)  [unwired: 7 in]
        n3341 = call "Write Instrument.lvclass.vi"("error in (no error)"=w8309, "Instrument.lvclass"=w8292, "S4ACS_GUI in"=w8294) -> ("error out"=w8288:errorcluster, "S4ACS_GUI out"=w8289:refnum<class "S4GUI.lvclass">)  [unwired: 7 in]
        n3342 = call "Read Instrument.lvclass.vi"("error in (no error)"=w8288, "S4ACS_GUI in"=w8289) -> ("error out"=w8359:errorcluster, "Instrument.lvclass"=w8360:refnum<class "Instrument.lvclass">, "S4ACS_GUI out"=w8200:refnum<class "S4GUI.lvclass">)  [unwired: 7 in]
        n3343 = call "Read WPSEL.vi"("error in (no error)"=w8359, "Instrument in"=w8360) -> ("error out"=w8356:errorcluster, "Opt_Selector.lvclass"=w8358:refnum<class "Opt_Selector.lvclass">, "Instrument out"=w8350:refnum<class "Instrument.lvclass">)  [unwired: 7 in]
        n3344 = call-dynamic "Read State Machine.vi"("error in (no error)"=w8356, "Device in"=w8358) -> ("error out"=w8355:errorcluster, "State Machine.lvclass"=w8348:refnum<class "State Machine.lvclass">, "Device out"=w8352:refnum<class "Opt_Selector.lvclass">)  [unwired: 7 in]
        n3345 = call "Next State.vi"("error in (no error)"=w8355, "New_State"=1, "State Machine in"=w8348) -> ("error out"=w8354:errorcluster, "State Machine out"=w8353:refnum<class "State Machine.lvclass">)  [unwired: 7 in]
        n3346 = call-dynamic "Write State Machine.vi"("error in (no error)"=w8354, "State Machine.lvclass"=w8353, "Device in"=w8352) -> ("error out"=w8349:errorcluster, "Device out"=w8351:refnum<class "Opt_Selector.lvclass">)  [unwired: 7 in]
        n3347 = call "Write WPSEL.vi"("error in (no error)"=w8349, "Opt_Selector.lvclass"=w8351, "Instrument in"=w8350) -> ("error out"=w8340:errorcluster, "Instrument out"=w8339:refnum<class "Instrument.lvclass">)  [unwired: 7 in]
        n3348 = call "Read ASEL.vi"("error in (no error)"=w8340, "Instrument in"=w8339) -> ("error out"=w8346:errorcluster, "Opt_Selector.lvclass"=w8337:refnum<class "Opt_Selector.lvclass">, "Instrument out"=w8338:refnum<class "Instrument.lvclass">)  [unwired: 7 in]
        n3349 = call-dynamic "Read State Machine.vi"("error in (no error)"=w8346, "Device in"=w8337) -> ("error out"=w8345:errorcluster, "State Machine.lvclass"=w8341:refnum<class "State Machine.lvclass">, "Device out"=w8336:refnum<class "Opt_Selector.lvclass">)  [unwired: 7 in]
        n3350 = call "Next State.vi"("error in (no error)"=w8345, "New_State"=1, "State Machine in"=w8341) -> ("error out"=w8344:errorcluster, "State Machine out"=w8343:refnum<class "State Machine.lvclass">)  [unwired: 7 in]
        n3351 = call-dynamic "Write State Machine.vi"("error in (no error)"=w8344, "State Machine.lvclass"=w8343, "Device in"=w8336) -> ("error out"=w8342:errorcluster, "Device out"=w8335:refnum<class "Opt_Selector.lvclass">)  [unwired: 7 in]
        n3352 = call "Write ASEL.vi"("error in (no error)"=w8342, "Opt_Selector.lvclass"=w8335, "Instrument in"=w8338) -> ("error out"=w8322:errorcluster, "Instrument out"=w8324:refnum<class "Instrument.lvclass">)  [unwired: 7 in]
        n3353 = call "Read CALW.vi"("error in (no error)"=w8322, "Instrument in"=w8324) -> ("error out"=w8332:errorcluster, "Opt_Selector.lvclass"=w8334:refnum<class "Opt_Selector.lvclass">, "Instrument out"=w8323:refnum<class "Instrument.lvclass">)  [unwired: 7 in]
        n3354 = call-dynamic "Read State Machine.vi"("error in (no error)"=w8332, "Device in"=w8334) -> ("error out"=w8331:errorcluster, "State Machine.lvclass"=w8325:refnum<class "State Machine.lvclass">, "Device out"=w8328:refnum<class "Opt_Selector.lvclass">)  [unwired: 7 in]
        n3355 = call "Next State.vi"("error in (no error)"=w8331, "New_State"=1, "State Machine in"=w8325) -> ("error out"=w8330:errorcluster, "State Machine out"=w8329:refnum<class "State Machine.lvclass">)  [unwired: 7 in]
        n3356 = property on="Lambda Selector" class="Ring (strict)"() -> ("RingText.Text"=w8321:string)  [unwired: 2 in, 2 out]
        n3357 = call-dynamic "Write State Machine.vi"("error in (no error)"=w8330, "State Machine.lvclass"=w8329, "Device in"=w8328) -> ("error out"=w8326:errorcluster, "Device out"=w8327:refnum<class "Opt_Selector.lvclass">)  [unwired: 7 in]
        n3358 = call "Write CALW.vi"("error in (no error)"=w8326, "Opt_Selector.lvclass"=w8327, "Instrument in"=w8323) -> ("error out"=w8199:errorcluster, "Instrument out"=w8320:refnum<class "Instrument.lvclass">)  [unwired: 7 in]
        n3359 = call-dynamic "Read mode EXPOSE.vi"("error in (no error)"=w8199, "S4GUI in"=w8200) -> ("error out"=w8198:errorcluster, "mode EXPOSE"=w8196:bool, "S4GUI out"=w8197:refnum<class "S4GUI.lvclass">)  [unwired: 7 in]
        n3360 = call-dynamic "Read sync.vi"("error in (no error)"=w8198, "S4ACS_GUI in"=w8197) -> ("error out"=w8219:errorcluster, "sync"=w8218:bool, "S4ACS_GUI out"=w8220:refnum<class "S4GUI.lvclass">)  [unwired: 7 in]
        n3361 = case shown="Default" w8321 {
          selector: w8321 -> [w8568 _]
          tunnel: w8320 -> [w8572 w8590]
          tunnel: [w8571 w8590] -> w8319
          tunnel: [w8564 w8589] -> w8236
          tunnel: w8219 -> [w8570 w8589]
          tunnel: [w8561 w8585] -> w8231
          tunnel: w8218 -> [w8560 _]
          tunnel: w8196 -> [w8559 w8588]
          frame "OFF" {
            w8562 = u16 0 items=["OFF", "POLARIZER", "PINHOLE", "SHUTTER", "DEPOLARIZER"] ("Calibrator Selector 2")
            n3362 = call "Read CALW.vi"("error in (no error)"=w8570, "Instrument in"=w8572) -> ("error out"=w8575:errorcluster, "Opt_Selector.lvclass"=w8577:refnum<class "Opt_Selector.lvclass">, "Instrument out"=w8576:refnum<class "Instrument.lvclass">)  [unwired: 7 in]
